vi "Helper - kph 2 mps.vi"(5 "km/hr":dbl) -> (2 "m/s":dbl)   [LabVIEW 2011]
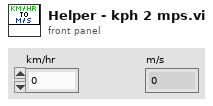
[diagram p1: front panel]
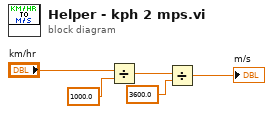
[diagram p0: block diagram]
diagram:
  n1 = Divide(x="km/hr", y=1000.0) -> (x/y=w2:dbl)
  n2 = Divide(x=w2, y=3600.0) -> (x/y=→"m/s":dbl)
